vi "Autonomous Independent.vi"   [LabVIEW 2014]
doc: "This VI is called when autonomous begins, and will automatically be terminated when autonomous ends. You can carry out timed or sensor driven robot movement independently without needing to return to the caller."
uses:
  <vilib>/Rock Robotics/WPI/Joystick/WPI_JoystickGetSetRefNum.vi
  Global Variables.vi
panel:
  # "Be sure to right-click and choose Data Operations>>Make Current Value default if you want to save the array values with the VI"
types:
  T1 = typedef "WPI_JoystickDevRef.ctl" = cluster{"Device":T2}
  T2 = typedef "WPI_JoystickDeviceEnum.ctl" = enum16{"USB 0", "USB 1", "USB 2", "USB 3", "USB 4", "USB 5"}
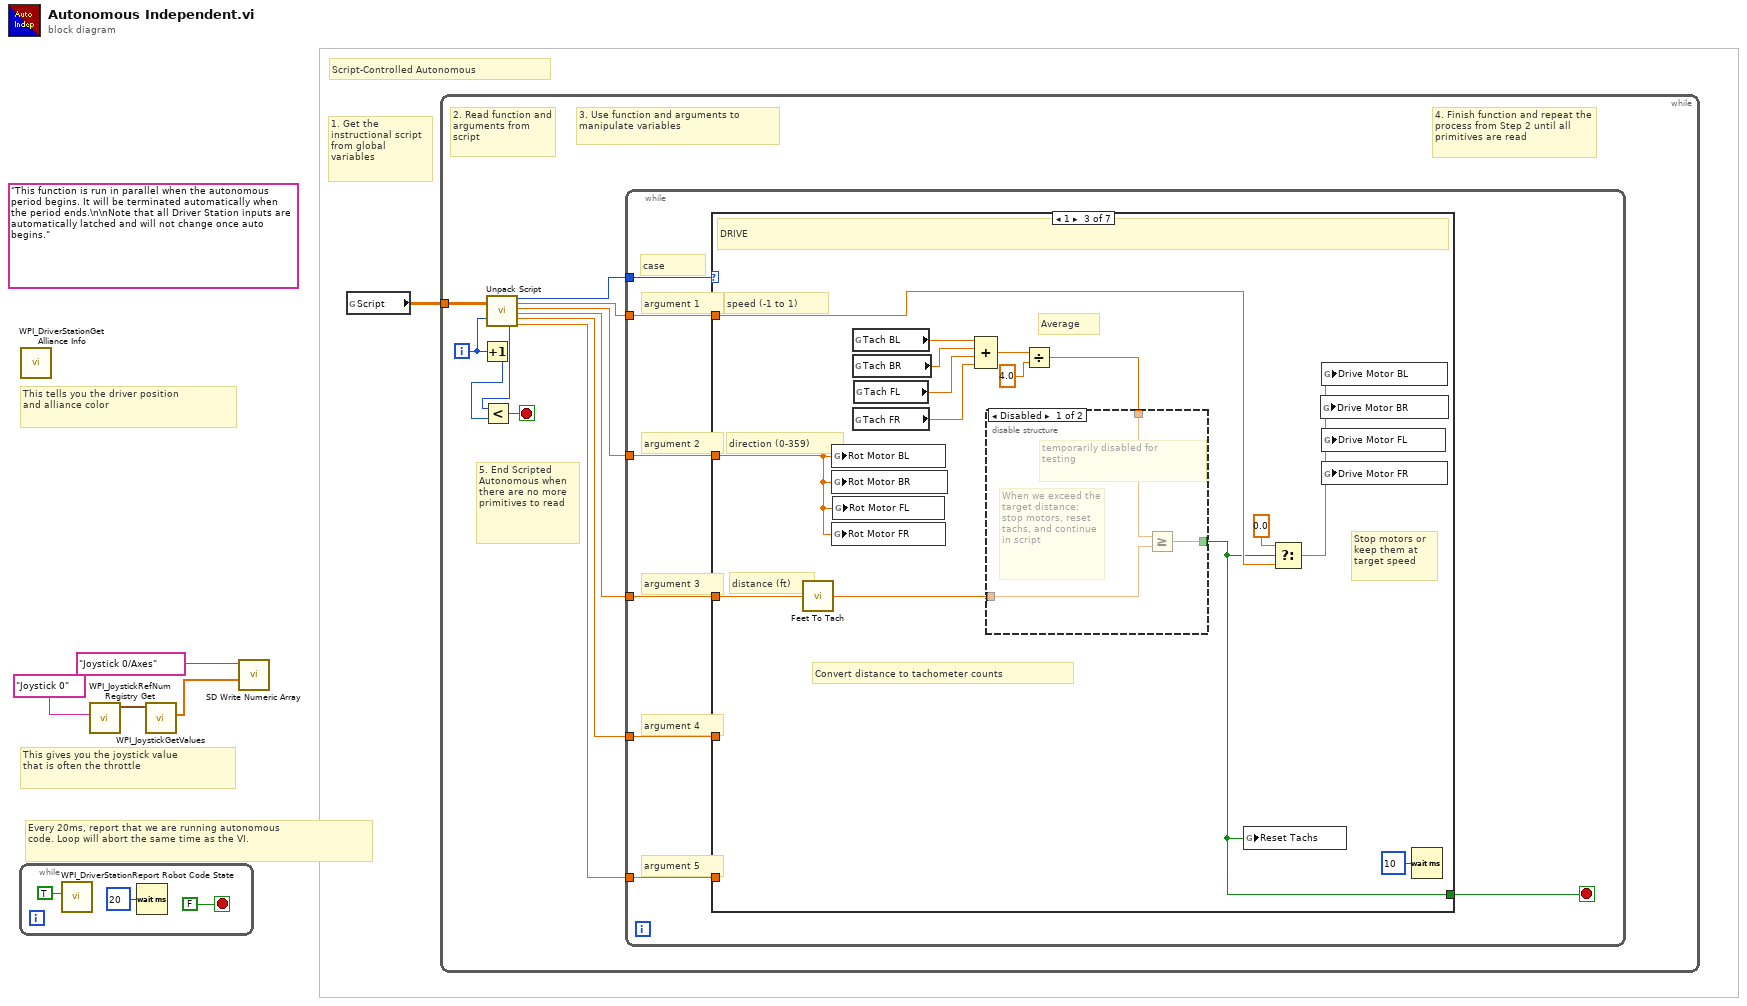
[diagram p0: block diagram]
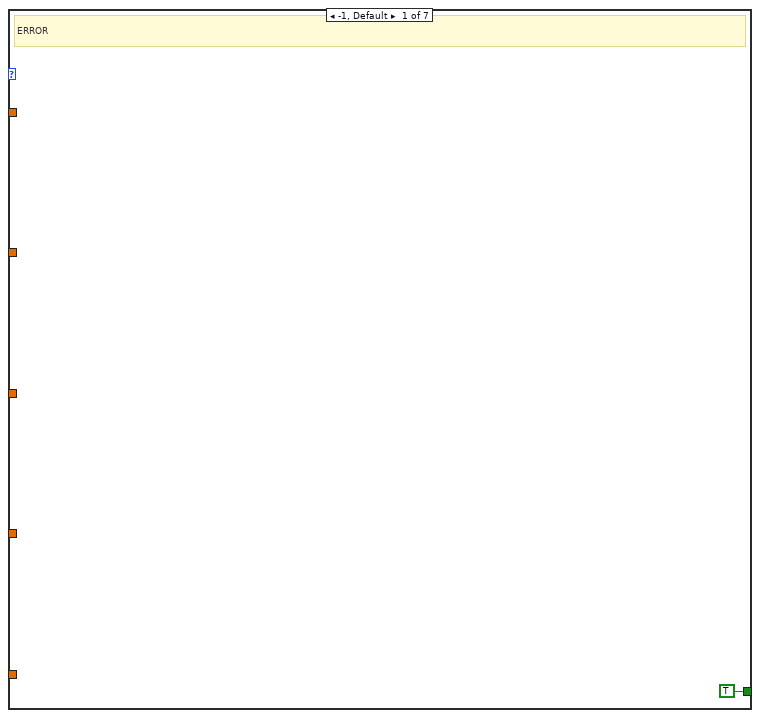
[diagram p2: hidden frame]
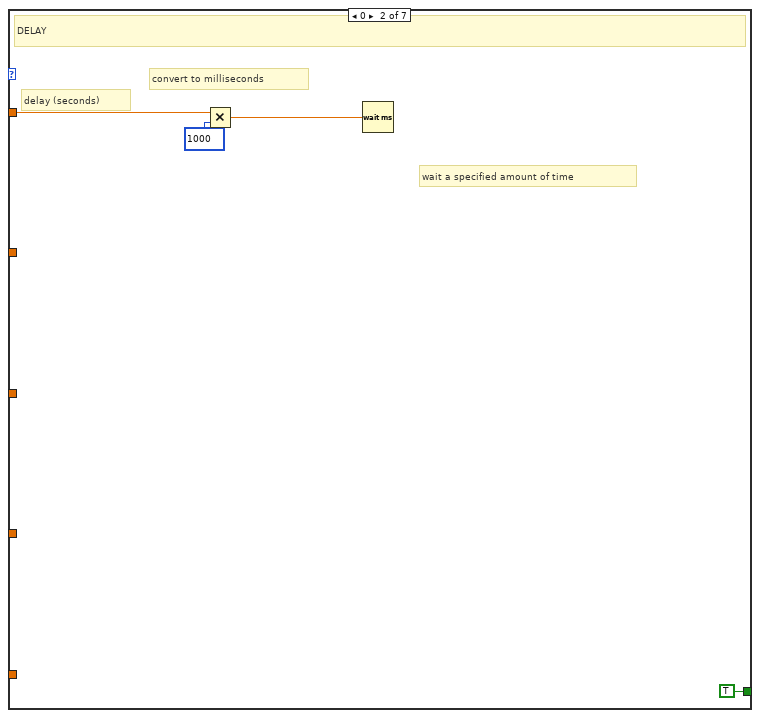
[diagram p3: hidden frame]
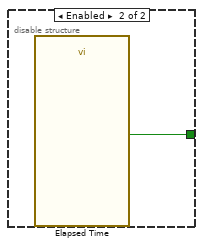
[diagram p4: hidden frame]
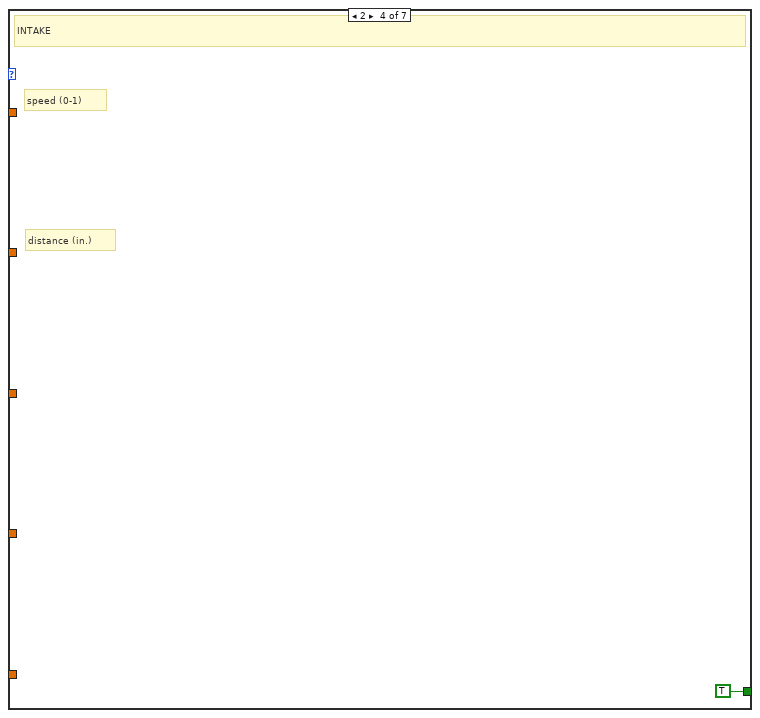
[diagram p5: hidden frame]
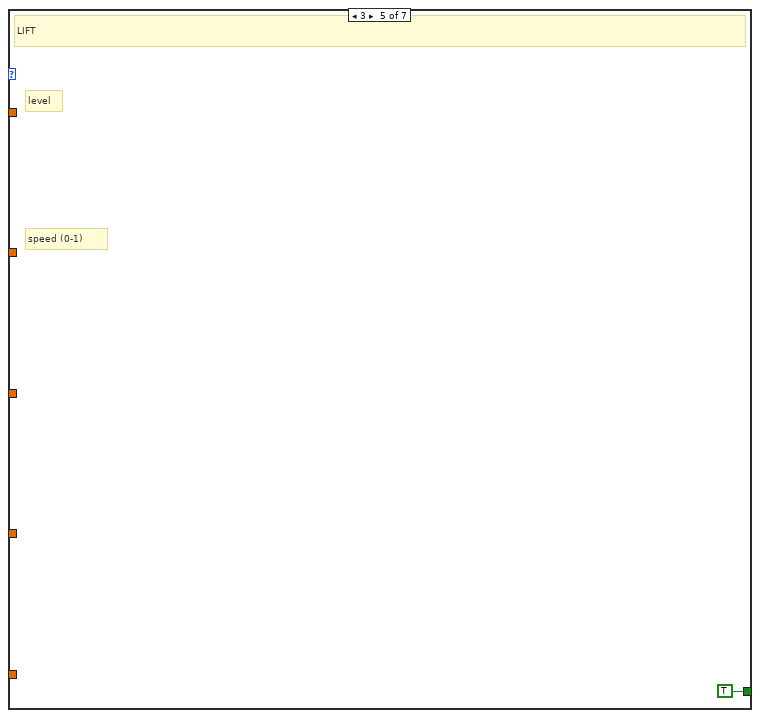
[diagram p6: hidden frame]
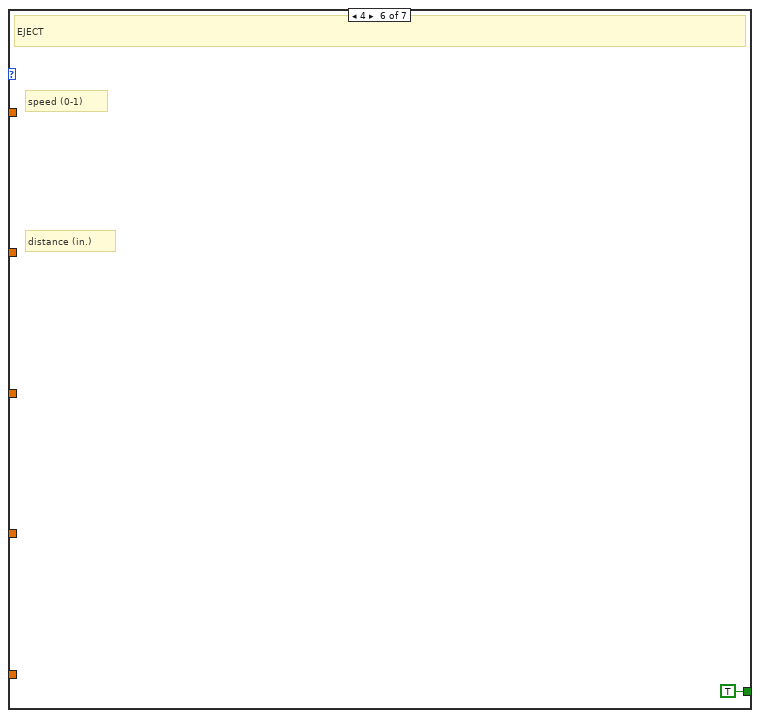
[diagram p7: hidden frame]
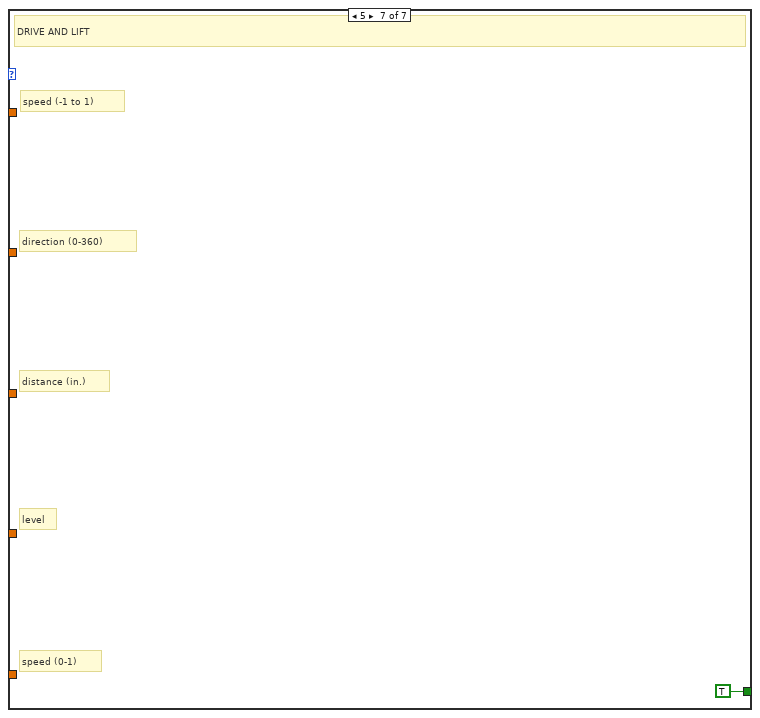
[diagram p8: hidden frame]
diagram:
  (unwired) "This function is run in parallel when the autonomous period begins. It will be terminated automatically when the period ends.\n\nNote that all Driver Station inputs are automatically latched and will not change once auto begins."
  # "1. Get the instructional script from global variables"
  # "Script-Controlled Autonomous"
  # "Every 20ms, report that we are running autonomous\ncode. Loop will abort the same time as the VI."
  # "This gives you the joystick value\nthat is often the throttle"
  # "This tells you the driver position\nand alliance color"
  n1 = while {
    stop <- FALSE stop-if-true
    n2 = call <vilib>:"WPI_DriverStationReport Robot Code State.vi"("Autonomous"=TRUE) -> ()  [unwired: 10 in, 1 out]
    n3 = Wait (ms)(milliseconds to wait=u32 20) -> ()  [unwired: 1 out]
  }
  n4 = call <vilib>:"WPI_DriverStationGet Alliance Info.vi"() -> ()  [unwired: 12 out]
  n5 = call <vilib>:"WPI_JoystickRefNum Registry Get.vi"("refnum name"="Joystick 0") -> ("JoystickDevRef"=w4:T1)  [unwired: 1 in, 9 out]
  n6 = call <vilib>:"WPI_JoystickGetValues.vi"("JoystickDevRef"=w4) -> ("Axes"=w2:dbl[])  [unwired: 6 in, 4 out]
  n7 = call <vilib>:"SD Write Numeric Array.vi"("Numeric Array"=w2, "Name"="Joystick 0/Axes") -> ()  [unwired: 8 in, 2 out]
  n8 = global read "Global Variables.vi" "Script"() -> (w1:dbl[][])
  n9 = while {
    tunnel: w1 -> [w9]
    i -> [w13]
    stop <- w19 stop-if-true
    # "4. Finish function and repeat the process from Step 2 until all primitives are read"
    # "3. Use function and arguments to manipulate variables"
    # "5. End Scripted Autonomous when there are no more primitives to read"
    # "2. Read function and arguments from script"
    n10 = Increment(x=w13) -> (x+1=w11:i32)
    n11 = call "Unpack Script.vi"("script"=w9, "index"=w13) -> ("# of primitives"=w10:i32, "primitive"=w12:i32, "argument 1"=w18:dbl, "argument 2"=w17:dbl, "argument 3"=w16:dbl, "argument 4"=w15:dbl, "argument 5"=w14:dbl)  [unwired: 11 in]
    n12 = Less?(x=w10, y=w11) -> (x < y?=w19:bool)
    n13 = while {
      tunnel: w18 -> [w26]
      tunnel: w17 -> [w25]
      tunnel: w16 -> [w24]
      tunnel: w15 -> [w23]
      tunnel: w14 -> [w22]
      tunnel: w12 -> [w21]
      stop <- w20 stop-if-true
      # "case"
      # "argument 5"
      # "argument 4"
      # "argument 3"
      # "argument 2"
      # "argument 1"
      n14 = case shown="1" w21 {
        tunnel: w26 -> [_ w30 w37 _ _ _ _]
        tunnel: w25 -> [_ _ w34 _ _ _ _]
        tunnel: w24 -> [_ _ w46 _ _ _ _]
        tunnel: w23 -> [_ _ _ _ _ _ _]
        tunnel: w22 -> [_ _ _ _ _ _ _]
        tunnel: [TRUE TRUE w32 TRUE TRUE TRUE TRUE] -> w20
        frame -1, Default {
          # "ERROR"
        }
        frame 0 {
          # "wait a specified amount of time"
          # "convert to milliseconds"
          # "delay (seconds)"
          # "DELAY"
          n15 = Multiply(x=w30, y=1000) -> (x*y=w29:dbl)
          n16 = Wait (ms)(milliseconds to wait=w29) -> ()  [unwired: 1 out]
        }
        frame 1 {
          # "Stop motors or keep them at target speed"
          # "Average"
          # "Convert distance to tachometer counts"
          # "distance (ft)"
          # "direction (0-359)"
          # "speed (-1 to 1)"
          # "DRIVE"
          n17 = call "Feet To Tach.vi"("Feet"=w46) -> ("Tach Counts"=w38:dbl)
          n18 = global write "Global Variables.vi" "Rot Motor BL"(w34) -> ()
          n19 = global write "Global Variables.vi" "Rot Motor BR"(w34) -> ()
          n20 = global write "Global Variables.vi" "Rot Motor FR"(w34) -> ()
          n21 = global write "Global Variables.vi" "Rot Motor FL"(w34) -> ()
          n22 = global read "Global Variables.vi" "Tach BL"() -> (w45:dbl)
          n23 = global read "Global Variables.vi" "Tach BR"() -> (w44:dbl)
          n24 = global read "Global Variables.vi" "Tach FR"() -> (w42:dbl)
          n25 = global read "Global Variables.vi" "Tach FL"() -> (w43:dbl)
          n26 = Compound Arithmetic op=ADD(w45, w44, w43, w42) -> (w41:dbl)
          n27 = Divide(x=w41, y=4.0) -> (x/y=w39:dbl)
          n28 = disable-structure shown="Disabled" {
            disable-tunnel: w39 -> [w49 _]
            disable-tunnel: w38 -> [w48 _]
            disable-tunnel: [w47 w50] -> w32
            frame Disabled {
              # "When we exceed the target distance: stop motors, reset tachs, and continue in script"
              # "temporarily disabled for\ntesting"
              n29 = Greater Or Equal?(x=w49, y=w48) -> (x >= y?=w47:bool)
            }
            frame Enabled {
              n30 = call "Elapsed Time"() -> ("Time has Elapsed"=w50:bool)  [unwired: 12 in, 7 out]
            }
          }
          n31 = global write "Global Variables.vi" "Reset Tachs"(w32) -> ()
          n32 = Select(t=0.0, s=w32, f=w37) -> (s? t:f=w35:dbl)
          n33 = global write "Global Variables.vi" "Drive Motor BR"(w35) -> ()
          n34 = global write "Global Variables.vi" "Drive Motor BL"(w35) -> ()
          n35 = global write "Global Variables.vi" "Drive Motor FL"(w35) -> ()
          n36 = global write "Global Variables.vi" "Drive Motor FR"(w35) -> ()
          n37 = Wait (ms)(milliseconds to wait=u32 10) -> ()  [unwired: 1 out]
        }
        frame 2 {
          # "distance (in.)"
          # "speed (0-1)"
          # "INTAKE"
        }
        frame 3 {
          # "speed (0-1)"
          # "level"
          # "LIFT"
        }
        frame 4 {
          # "distance (in.)"
          # "speed (0-1)"
          # "EJECT"
        }
        frame 5 {
          # "speed (0-1)"
          # "level"
          # "distance (in.)"
          # "direction (0-360)"
          # "speed (-1 to 1)"
          # "DRIVE AND LIFT"
        }
      }
    }
  }
